vi "send serial command tester no visa.vi"(7 "time (s)":dbl, 8 "error in (no error)":errorcluster, 9 "data":dbl[](array[numeric]), 10 "Command":T1, 11 "visa resource":refnum<visa-resource-name>) -> (0 "error out":errorcluster, 2 "command string":string, 3 "VISA resource name out":refnum<visa-resource-name>)   [LabVIEW 2020]
uses:
  typedefs/commandType.ctl
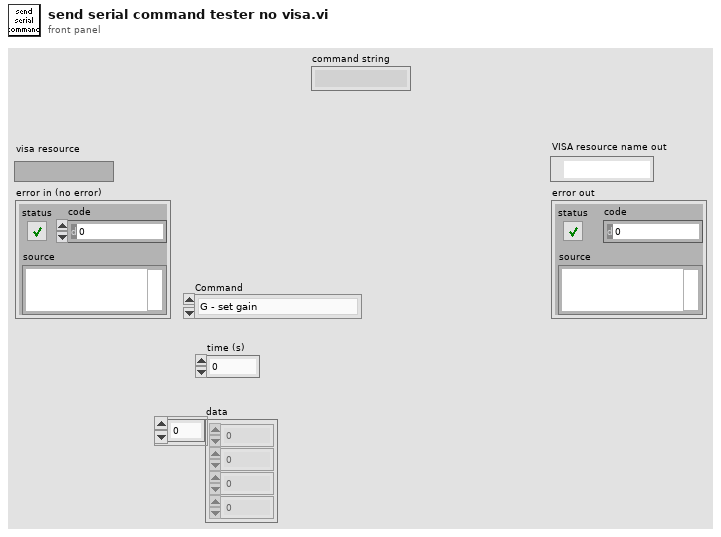
[diagram p1: front panel]
types:
  T1 = typedef "commandType.ctl" = enum16{"G - set gain", "C - activate coil", "D - deactivate coil", "L - set LED", "A - set AUTO", "V - set verbose", "T - set transmission", "R - get version", "Z - zero accelerometer", "F - set auto-flash led", "X - synchronize serial", "Q - reset queues and timers", "S - save configuration"}
  T2 = cluster{"data[0]":dbl, "data[1]":dbl, "data[2]":dbl, "data[3]":dbl}
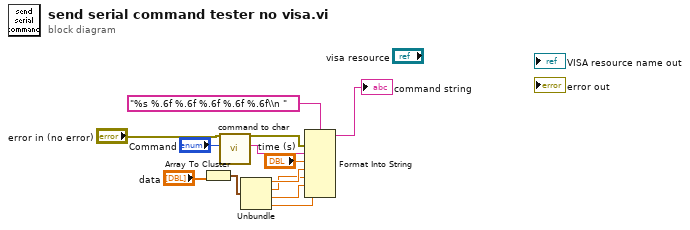
[diagram p0: block diagram]
diagram:
  n1 = Array To Cluster(array="data") -> (cluster=w9:T2)
  n2 = call "command to char.vi"("Command"="Command") -> ("char"=w12:string)  [unwired: 10 in]
  n3 = Unbundle(w9) -> ("data[0]"=w8:dbl, "data[1]"=w7:dbl, "data[2]"=w6:dbl, "data[3]"=w5:dbl)
  n4 = Format Into String(format string="%s %.6f %.6f %.6f %.6f %.6f\\n ", error in="error in (no error)", w12, "time (s)", w8, w7, w6, w5) -> (resulting string=→"command string":string, error out=w2:errorcluster)  [unwired: 1 in]
